vi "Bloques.vi"() -> ()   [LabVIEW 2020]
panel:
  in  "?":bool
  out "Waveform Graph":dynamicdata(graph)
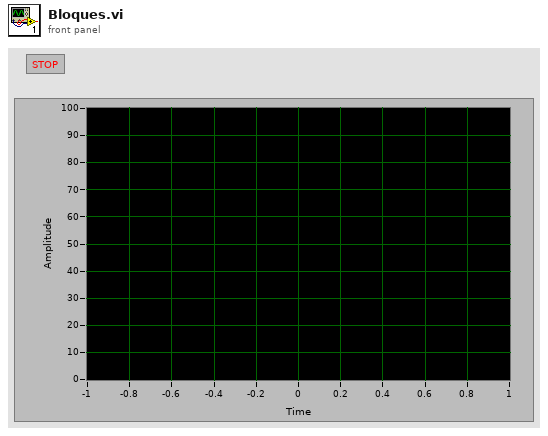
[diagram p1: front panel]
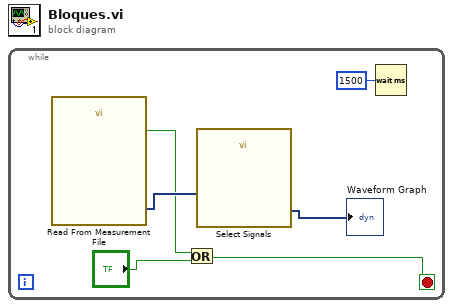
[diagram p0: block diagram]
diagram:
  n1 = while {
    stop <- w1 stop-if-true
    n2 = call "Read From Measurement File"() -> ("Signals"=w4:dynamicdata, "EOF?"=w2:bool)  [unwired: 6 in, 4 out]
    n3 = Or(x=w2, y="?") -> (x .or. y?=w1:bool)
    n4 = call "Select Signals"("Signals"=w4) -> ("Signal Out"=→"Waveform Graph":dynamicdata)  [unwired: 9 in, 1 out]
    n5 = Wait (ms)(milliseconds to wait=1500) -> ()  [unwired: 1 out]
  }
